vi "PRL BUFFER Rearrange Digital 2D Array.vi"(10 "Cut Index":i32, 11 "Array In":bool[][](array[boolean])) -> (3 "Array Out":bool[][](array[boolean]))   [LabVIEW 2013, in "PMU Recorder Light.lvlib"]
uses:
  PMU Recorder Light.lvlib
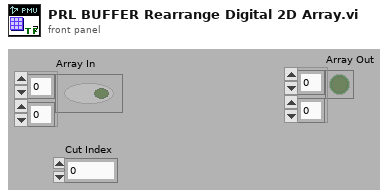
[diagram p1: front panel]
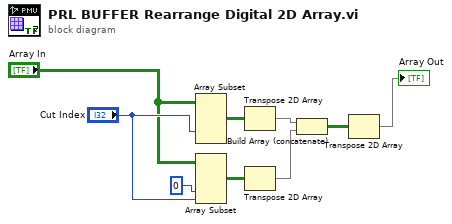
[diagram p0: block diagram]
diagram:
  n1 = Array Subset(array="Array In", index (col)="Cut Index") -> (w9:bool[][])  [unwired: 3 in]
  n2 = Array Subset(array="Array In", index (col)=0 ("index"), length (col)="Cut Index") -> (w8:bool[][])  [unwired: 2 in]
  n3 = Transpose 2D Array(2D array=w9) -> (transposed array=w3:bool[][])
  n4 = Transpose 2D Array(2D array=w8) -> (transposed array=w2:bool[][])
  n5 = Build Array (concatenate)(w3, w2) -> (w4:bool[][])
  n6 = Transpose 2D Array(2D array=w4) -> (transposed array=→"Array Out":bool[][])
